vi "Create I32Message.vi"(8 "error in (no error)":errorcluster, 10 "Message Data":i32, 11 "Message Name":string) -> (0 "error out":errorcluster, 3 "I32Message out":refnum<class "I32Message.lvclass">)   [LabVIEW 2009, in "LapDog.Messaging.v2.NativeTypes.lvlib" / "I32Message.lvclass"]
doc: "Returns an I32Message object with the given name.\n\nThis method executes regardless of the error in state."
uses:
  I32Message.lvclass
  I32Message.lvclass/I32Message.ctl
  Messaging.v2/MessageObject/Message.lvclass
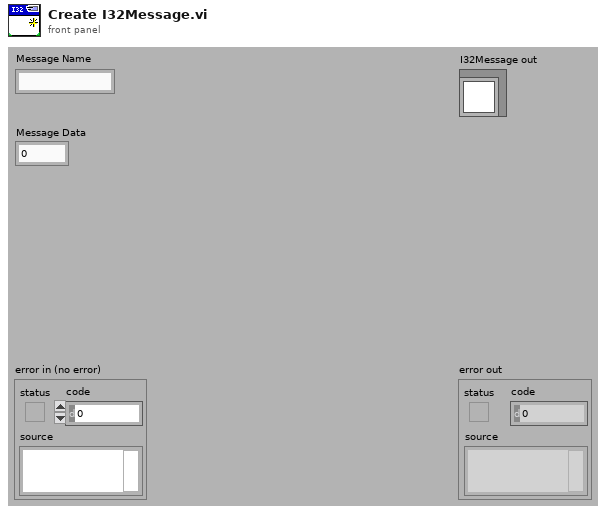
[diagram p1: front panel]
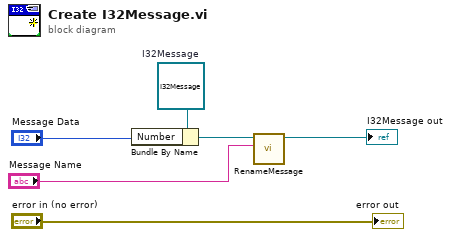
[diagram p0: block diagram]
diagram:
  w6 = refnum<class "I32Message.lvclass"> refnum  # I32Message
  n1 = Bundle By Name(cluster=w6, "Number"="Message Data") -> (w3:refnum<class "I32Message.lvclass">)
  n2 = call "RenameMessage.vi"("Message Name"="Message Name", "Message in"=w3) -> ("Message out"=→"I32Message out":refnum<class "I32Message.lvclass">)  [unwired: 8 in, 1 out]
  "error out" <- "error in (no error)"
